vi "IMAQ Test 11_27_17.vi"() -> ()   [LabVIEW 2012]
uses:
  <vilib>/userdefined/High Color/IMAQdx.ctl
  <vilib>/vision/driver/NI_Vision_Acquisition_Software.lvlib
panel:
  out "error out 4":errorcluster
  in  "Take Image":bool
  out "error out 3":errorcluster
  out "error out 2":errorcluster
  in  "stop":bool
  out "?":T1(plugin-control)
  out "error out":errorcluster
  in  "Session In":T2
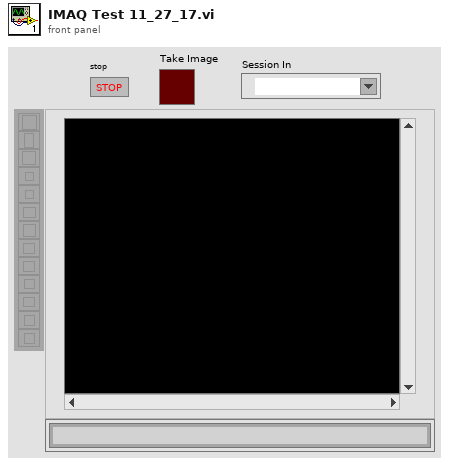
[diagram p1: front panel]
types:
  T1 = typedef "IMAQ Image.ctl" = refnum<image>
  T2 = typedef "IMAQdx.ctl" = refnum<k21>
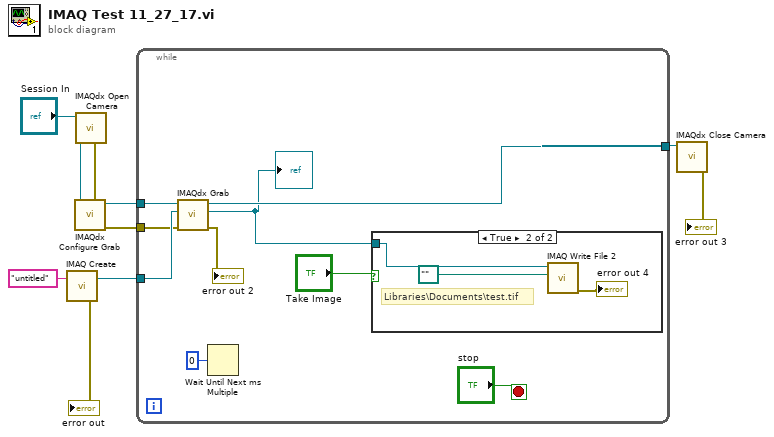
[diagram p0: block diagram]
diagram:
  n1 = call "IMAQ Create"("Image Name"="untitled") -> ("New Image"=w6:T1, "error out"=→"error out":errorcluster)  [unwired: 4 in]
  n2 = call <vilib>:"IMAQdx Open Camera.vi"("Session In"="Session In") -> ("error out"=w8:errorcluster, "Session Out"=w9:T2)  [unwired: 9 in]
  n3 = call <vilib>:"IMAQdx Configure Grab.vi"("error in"=w8, "Session In"=w9) -> ("error out"=w2:errorcluster, "Session Out"=w7:T2)  [unwired: 8 in]
  n4 = while {
    tunnel: w7 -> [w19]
    tunnel: w6 -> [w18]
    tunnel: [w17] -> w3
    tunnel: w2 -> [w15]
    stop <- "stop" stop-if-true
    n5 = call <vilib>:"IMAQdx Grab.vi"("error in"=w15, "Image In"=w18, "Session In"=w19) -> ("error out"=→"error out 2":errorcluster, "Image Out"=w11:T1, "Session Out"=w17:T2)  [unwired: 5 in, 1 out]
    "?" <- w11
    n6 = Wait Until Next ms Multiple(millisecond multiple=u32 0) -> ()  [unwired: 1 out]
    n7 = case shown="True" "Take Image" {
      tunnel: w11 -> [_ w22]
      frame False {
      }
      frame True {
        # "Libraries\\Documents\\test.tif"
        n8 = call-poly "IMAQ Write File 2"("File Path"=path "", "Image"=w22) -> ("error out"=→"error out 4":errorcluster)  [unwired: 8 in, 1 out]
      }
    }
  }
  n9 = call <vilib>:"IMAQdx Close Camera.vi"("Session In"=w3) -> ("error out"=→"error out 3":errorcluster)  [unwired: 10 in]
